vi "Read.vi"(0 "VISA resource name":refnum<visa-resource-name>="GPIB0::23::INSTR", 11 "error in (no error)":errorcluster) -> (4 "VISA resource name out":refnum<visa-resource-name>, 8 "double precision float":dbl, 15 "error out":errorcluster)   [LabVIEW 2013, in "Stanford Research CG635.lvlib"]
uses:
  <instrlib>/Stanford Research CG635/Stanford Research CG635.lvlib
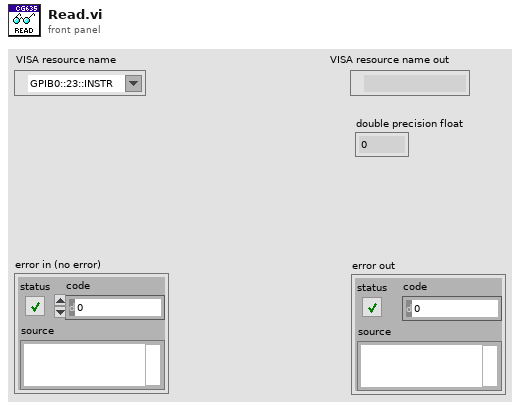
[diagram p1: front panel]
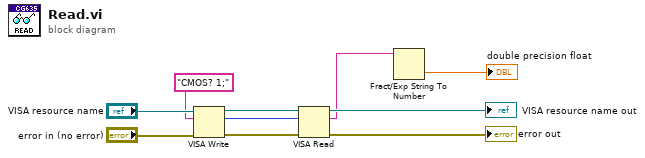
[diagram p0: block diagram]
diagram:
  n1 = VISA Write(VISA resource name="VISA resource name", write buffer="CMOS? 1;", error in (no error)="error in (no error)") -> (VISA resource name out=w6:refnum<visa-resource-name>, return count=w7:u32, error out=w5:errorcluster)
  n2 = VISA Read(VISA resource name=w6, byte count=w7, error in (no error)=w5) -> (VISA resource name out=→"VISA resource name out":refnum<visa-resource-name>, read buffer=w2:string, error out=→"error out":errorcluster)  [unwired: 1 out]
  n3 = Fract/Exp String To Number(string=w2) -> (number=→"double precision float":dbl)  [unwired: 3 in, 1 out]
